vi "autoninfo.vi"() -> ()   [LabVIEW 2019]
doc: "These global variables report autonomous sequencing and path following data."
panel:
  out "Auto_Spin_Shooter":bool
  out "Auto_Force_To_Low_Gear":bool
  out "Auto_Path_Suffix":string
  out "Auto_Error":errorcluster
  out "Distance_From_Start (in)":dbl
  out "Distance_From_End (in)":dbl
  out "Auto_Manipulator_Step":i32
  out "Auto_Drive_Step":i32
  out "Auto_Manipulator_Action":string
  out "Auto_Drive_Action":string
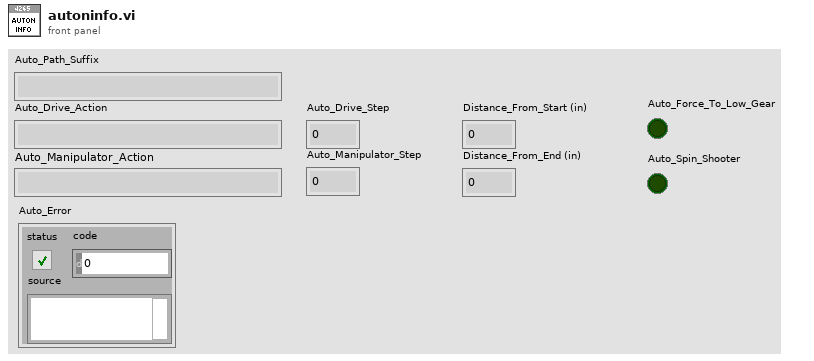
[diagram p1: front panel]
diagram:
